vi "set_config_cluster.vi"(8 "error in (no error)":errorcluster, 10 "config cluster variant":variant, 11 "FPGAWrapperMH120124FrameScan_PXI7813R in":refnum<class "FPGAWrapperMH120124FrameScan_PXI7813R.lvclass">) -> (0 "error out":errorcluster, 3 "FPGAWrapperMH120124FrameScan_PXI7813R out":refnum<class "FPGAWrapperMH120124FrameScan_PXI7813R.lvclass">)   [LabVIEW 2010, in "FPGAWrapperMH120124FrameScan_PXI7813R.lvclass"]
uses:
  FPGAWrapperMH120124FrameScan_PXI7813R.lvclass
  FPGAWrapperMH120124FrameScan_PXI7813R.lvclass/FPGAWrapperMH120124FrameScan_PXI7813R.ctl
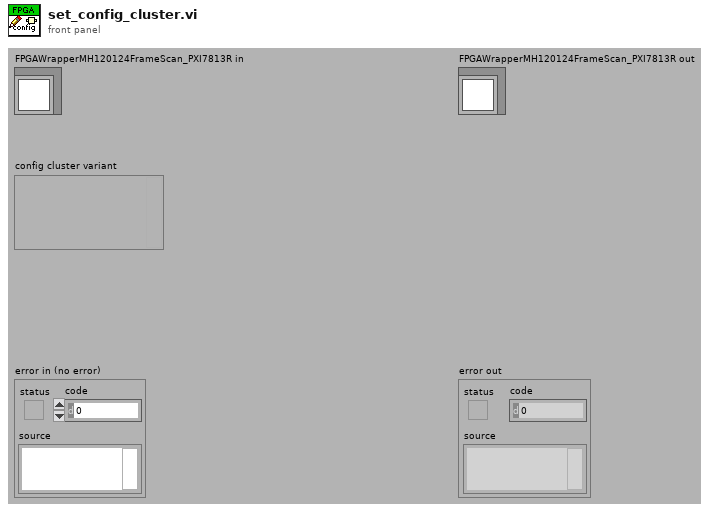
[diagram p1: front panel]
types:
  T1 = typedef "configuration_cluster_framescan.ctl" = cluster{"DDS board initialization parameters":T2, "inverse?":enum16{"normal", "x inversed", "y inversed", "x & y inversed"}, "OSK select":bool, "AOD equilibration time":dbl[unit], "AOD amplitude":dbl, "AOD center frequ. (Hz)":dbl[unit], "AOD Bandwidth":dbl[unit], "FPGA wrapper path":string}
  T2 = typedef "DDS_board_init_cluster.ctl" = cluster{"Bypass PLL":bool, "PLL Range":bool, "Update Clock":bool, "Triangle ":bool, "SDO Active":bool, "LSB First":bool, "OSK Int":bool, "Output Shaped Keying Enable":bool, "Bypass Sinc":bool, "Digital Part":bool, "OutPut DAC":bool, "Control DAC":bool, "Comparator":bool, "Modus":u8, "Multiplier Value":u8}
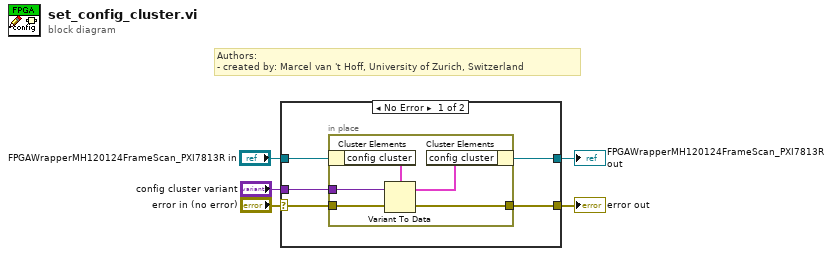
[diagram p0: block diagram]
diagram:
  # "Authors: \n- created by: Marcel van 't Hoff, University of Zurich, Switzerland"
  n1 = case shown="No Error" "error in (no error)" {
    selector: "error in (no error)" -> [w7 w17]
    tunnel: [w6 w17] -> w4
    tunnel: [w8 w16] -> w3
    tunnel: "FPGAWrapperMH120124FrameScan_PXI7813R in" -> [w9 w16]
    tunnel: "config cluster variant" -> [w10 _]
    frame No Error {
      n2 = in-place {
        in-place-border: w10 -> [w15]
        in-place-border: w7 -> [w14]
        in-place-border: [w13] -> w6
        n3 = in-place-cluster #1(w9) -> ("config cluster"=w12:T1)
        n4 = Variant To Data(error in=w14, Variant=w15, type=w12) -> (error out=w13:errorcluster, data=w11:T1)
        n5 = in-place-cluster #1("config cluster"=w11) -> (w8:refnum<class "FPGAWrapperMH120124FrameScan_PXI7813R.lvclass">)
      }
    }
    frame Error {
    }
  }
  "error out" <- w4
  "FPGAWrapperMH120124FrameScan_PXI7813R out" <- w3
